vi "Live File Test.vi"() -> ()   [LabVIEW 2021]
uses:
  Live File States.ctl
panel:
  in  "stop":bool
  in  "Refresh time (s)":dbl=1.0 caption="Delay Time (s)"
  out "File Contents":string
  in  "file path (use dialog)":path
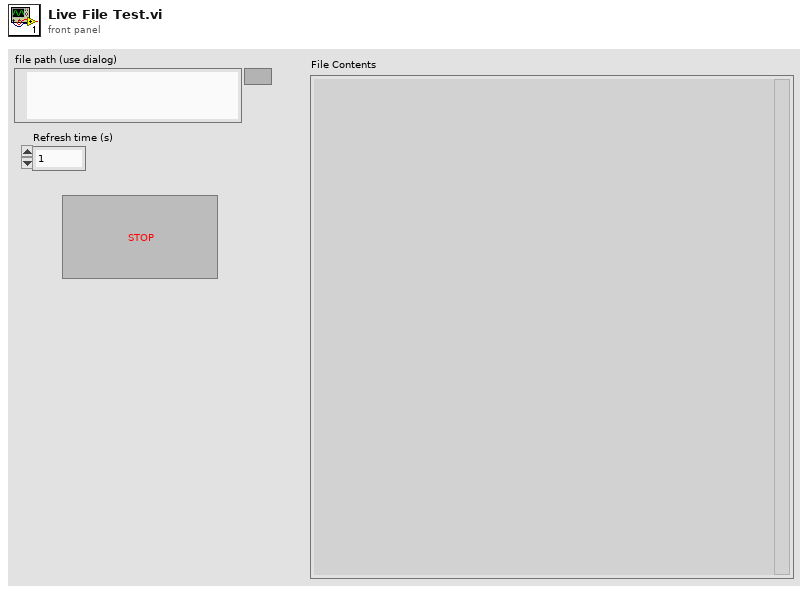
[diagram p1: front panel]
types:
  T1 = typedef "Live File States.ctl" = enum16{"Init & Open File", "Check & Update", "Exit"}
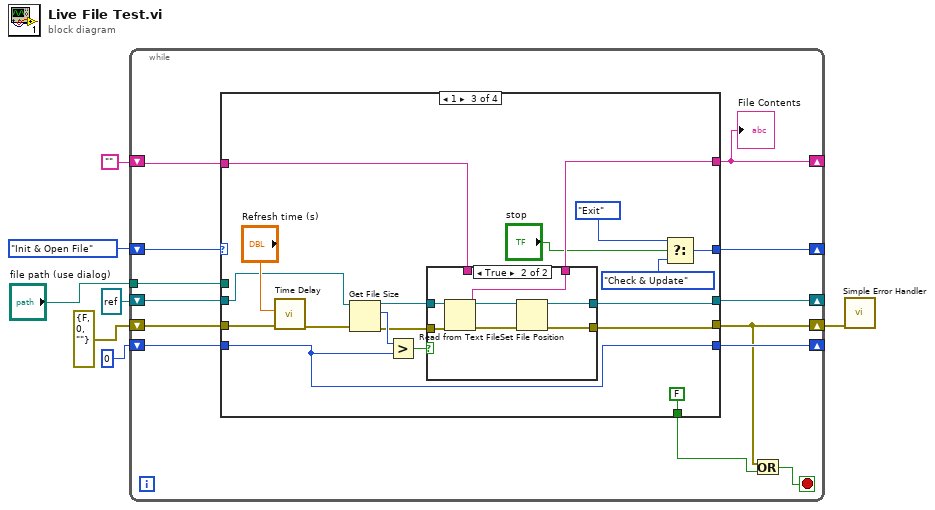
[diagram p0: block diagram]
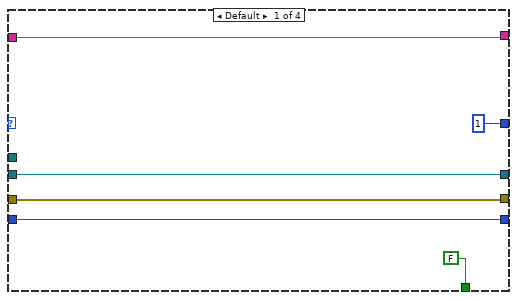
[diagram p2: hidden frame]
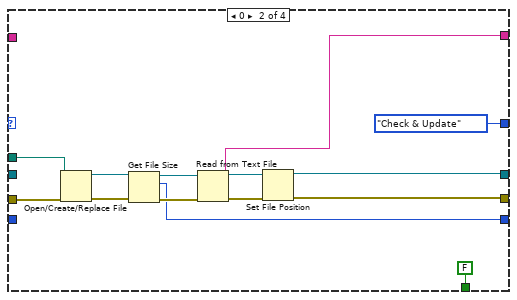
[diagram p3: hidden frame]
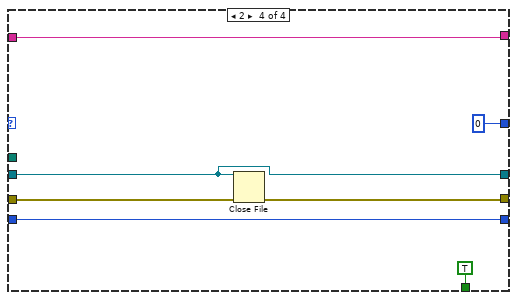
[diagram p5: hidden frame]
diagram:
  n1 = while {
    shift-right: [w20] -> _
    shift-left: Live_File_States."Init & Open File" -> [w11]
    tunnel: "file path (use dialog)" -> [w19]
    shift-right: [w10] -> w1
    shift-left: errorcluster {"status"=FALSE, "code"=0, "source"=""} ("error out") -> [w18]
    shift-right: [w17] -> _
    shift-left: refnum<file> refnum ("refnum out") -> [w15]
    shift-right: [w16] -> _
    shift-left: "" -> [w12]
    shift-right: [w14] -> _
    shift-left: i64 0 ("size (in bytes)") -> [w13]
    stop <- w8 stop-if-true
    n2 = case shown="1" w11 {
      tunnel: [u16 1 ("f") Live_File_States."Check & Update" w43 u16 0 ("f")] -> w20
      tunnel: w19 -> [_ w40 _ _]
      tunnel: [w24 w27 w49 w69] -> w10
      tunnel: w18 -> [w24 w39 w57 w71]
      tunnel: [w25 w28 w47 w70] -> w17
      tunnel: [w26 w38 w48 w72] -> w16
      tunnel: w15 -> [w25 _ w55 w70]
      tunnel: [w23 w32 w52 w74] -> w14
      tunnel: w13 -> [w23 _ w52 w74]
      tunnel: w12 -> [w26 _ w46 w72]
      tunnel: [FALSE FALSE FALSE TRUE] -> w9
      frame Default {
      }
      frame 0 {
        n3 = Open/Create/Replace File(file path (use dialog)=w40, error in=w39) -> (refnum out=w35:refnum<file>, error out=w36:errorcluster)  [unwired: 4 in, 1 out]
        n4 = Get File Size(file=w35, error in=w36) -> (refnum out=w34:refnum<file>, size (in bytes)=w32:i64, 0:w33:errorcluster)
        n5 = Read from Text File(file (use dialog)=w34, error in=w33) -> (refnum out=w30:refnum<file>, text=w38:string, error out=w29:errorcluster)  [unwired: 2 in, 1 out]
        n6 = Set File Position(refnum=w30, error in=w29) -> (refnum out=w28:refnum<file>, error out=w27:errorcluster)  [unwired: 2 in]
      }
      frame 1 {
        n7 = call "Time Delay"("error in (no error)"=w57, "Delay Time (s)"="Refresh time (s)") -> ("error out"=w56:errorcluster)  [unwired: 9 in]
        n8 = Get File Size(file=w55, error in=w56) -> (refnum out=w50:refnum<file>, size (in bytes)=w54:i64, 0:w51:errorcluster)
        n9 = Greater?(x=w54, y=w52) -> (0:w53:bool)
        n10 = case shown="True" w53 {
          tunnel: w51 -> [w61 w68]
          tunnel: w50 -> [w60 w67]
          tunnel: [w61 w62] -> w49
          tunnel: [w59 w66] -> w48
          tunnel: [w60 w63] -> w47
          tunnel: w46 -> [w59 _]
          frame False {
          }
          frame True {
            n11 = Read from Text File(file (use dialog)=w67, error in=w68) -> (refnum out=w65:refnum<file>, text=w66:string, error out=w64:errorcluster)  [unwired: 2 in, 1 out]
            n12 = Set File Position(refnum=w65, error in=w64) -> (refnum out=w63:refnum<file>, error out=w62:errorcluster)  [unwired: 2 in]
          }
        }
        n13 = Select(t=Live_File_States."Exit", s="stop", f=Live_File_States."Check & Update") -> (s? t:f=w43:T1)
      }
      frame 2 {
        n14 = Close File(refnum=w70, error in=w71) -> (error out=w69:errorcluster)  [unwired: 1 out]
      }
    }
    "File Contents" <- w16
    n15 = Or(x=w10, y=w9) -> (x .or. y?=w8:bool)
  }
  n16 = call <vilib>:"Simple Error Handler.vi"("error in (no error)"=w1) -> ()  [unwired: 4 in, 5 out]
